vi "Gasauswahl befuellen.vi"(11 "Kombinationsfeld (Eingang)":refnum<vi>) -> ()   [LabVIEW 2020, in "System Einstellungen V2.lvlib"]
uses:
  System Einstellungen V2.lvlib
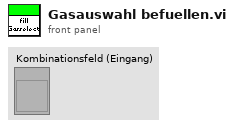
[diagram p1: front panel]
types:
  T1 = enum16{"lesen", "schreiben", "löschen", "laden", "speichern"}
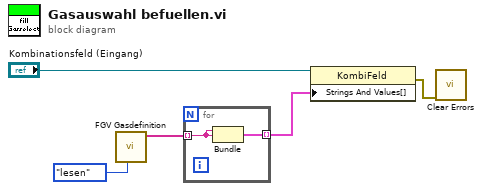
[diagram p0: block diagram]
diagram:
  n1 = call "FGV Gasdefinition.vi"("Aktion"=T1."lesen") -> ("Gase"=w2:string[])  [unwired: 9 in, 1 out]
  n2 = for {
    tunnel: w2 -> [w7] mode=indexing
    tunnel: [w6] -> w1 mode=indexing
    n3 = Bundle("Gas"=w7, "Gas"=w7) -> (w6:cluster{"Gas":string, "Gas":string})  [unwired: 1 in]
  }
  n4 = property class="KombiFeld"(reference="Kombinationsfeld (Eingang)", "Strings And Values[]"=w1) -> (error out=w5:errorcluster)  [unwired: 1 in, 1 out]
  n5 = call <vilib>:"Clear Errors.vi"("error in (no error)"=w5) -> ()  [unwired: 5 in, 2 out]
